vi "随机数发生器（乘同余法）.vi"(4 "X0":i32=11) -> (1 "Xi+1":i32)   [LabVIEW 2011]
doc: "功能：\n\n产生0-32768之间的随机整数。\n\n基本算法：\n\n使用同乘余法。\n\ncsxcs_366创建"
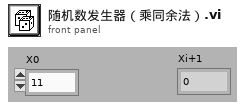
[diagram p1: front panel]
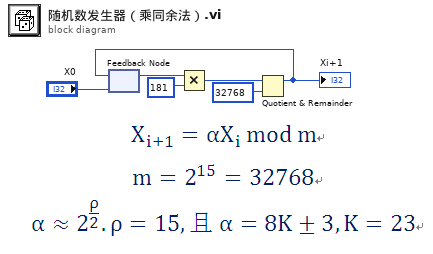
[diagram p0: block diagram]
diagram:
  n1 = feedback #1("X0") -> (w6:i32)
  n2 = Multiply(x=w6, y=181) -> (x*y=w4:i32)
  n3 = Quotient & Remainder(x=w4, y=32768) -> (x-y*floor(x/y)=w2:i32)  [unwired: 1 out]
  "Xi+1" <- w2
  n4 = feedback-in #1(w2) -> ()
